vi "Potting Data - HV Points.vi"(10 "HV Point Selection":bool[](array[boolean]), 11 "HV Point Data":T2[](array[typedef])) -> (3 "HV Potting Points":T1[](array[typedef]))   [LabVIEW 2011]
uses:
  Shared Components/Utils/Type Definitions/Fiducial Image.ctl
  Shared Components/Vec3d Class/Vec3d Class.lvclass
  Shared Components/Utils/Type Definitions/Physical Image.ctl
  <vilib>/vision/Image Controls.llb/IMAQ Image.ctl
  Shared Components/Utils/Type Definitions/Fiducial with Source.ctl
  Shared Components/Utils/Type Definitions/3d Point.ctl
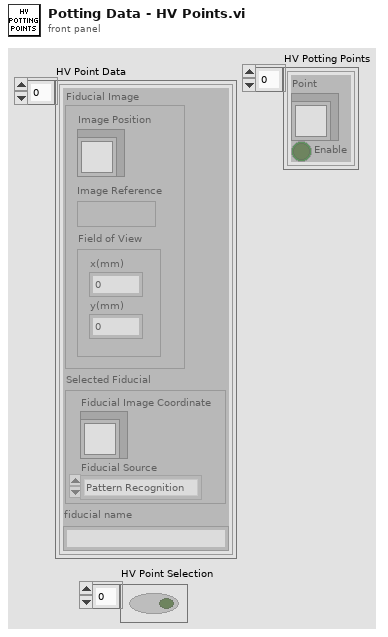
[diagram p1: front panel]
types:
  T1 = typedef "3d Point.ctl" = cluster{"Point":refnum<class "Vec3d Class.lvclass">, "Enable":bool}
  T2 = typedef "Fiducial Image.ctl" = cluster{"Fiducial Image":T3, "Selected Fiducial":T5, "fiducial name":string}
  T3 = typedef "Physical Image.ctl" = cluster{"Image Position":refnum<class "Vec3d Class.lvclass">, "Image Reference":T4, "Field of View":cluster{"x(mm)":dbl, "y(mm)":dbl}}
  T4 = typedef "IMAQ Image.ctl" = refnum<image>
  T5 = typedef "Fiducial with Source.ctl" = cluster{"Fiducial Image Coordinate":refnum<class "Vec3d Class.lvclass">, "Fiducial Source":enum16{"Pattern Recognition", "User", "Error", "Default"}}
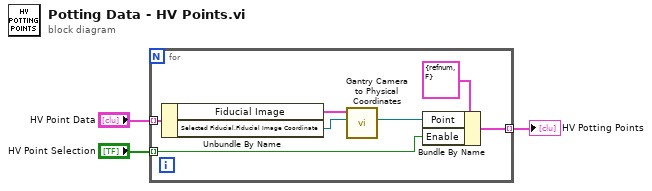
[diagram p0: block diagram]
diagram:
  n1 = for {
    tunnel: "HV Point Data" -> [w10] mode=indexing
    tunnel: "HV Point Selection" -> [w5] mode=indexing
    tunnel: [w4] -> w1 mode=indexing
    n2 = Unbundle By Name(w10) -> ("Fiducial Image"=w9:T3, "Selected Fiducial.Fiducial Image Coordinate"=w8:refnum<class "Vec3d Class.lvclass">)
    n3 = call "Gantry Camera to Physical Coordinates.vi"("Image Coordinate"=w8, "Physical Image"=w9) -> ("Global Coordinate"=w6:refnum<class "Vec3d Class.lvclass">)  [unwired: 7 in, 2 out]
    n4 = Bundle By Name(cluster=T1 {"Point"=refnum, "Enable"=FALSE} ("3d Point"), "Point"=w6, "Enable"=w5) -> (w4:T1)
  }
  "HV Potting Points" <- w1
